vi "Untitled 1.vi"   [LabVIEW 2016]
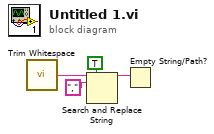
[diagram p0: block diagram]
diagram:
  n1 = call <vilib>:"Trim Whitespace.vi"() -> ("trimmed string"=w4:string)  [unwired: 2 in]
  n2 = Search and Replace String(replace all?=TRUE ("replace all? (F)"), input string=w4, search string=",") -> (result string=w1:string)  [unwired: 5 in, 3 out]
  n3 = Empty String/Path?(string/path=w1) -> ()  [unwired: 1 out]
